vi "FABR-Save Data.vi"(0 "Params":T3={"Stimulus"={"Destination"="", "Rep rate (/sec)"=30.0, "Alternate Polarity"=FALSE, "Duration (ms)"=0.0, "Ramp (ms)"=16.0, "Fs (Hz)"=5.0, "Frame size (s)"=0.0}, "Sequence"={"Freq"={"Start (kHz)"=20.0, "Stop (kHz)"=80.0, "Step (oct)"=5.0, "Skip (oct)"=0.0}, "Level"={"Start (dB)"=20, "Stop (dB)"=80, "Step (dB)"=5}, "Order"=enum."Interleaved"}, "Response"={"Gain"=1.0, "Averages"=0, "Window (ms)"=0.0, "Fs (Hz)"=25000.0, "Save raw"=FALSE}, "Reject"=0.0} {"Sequence"."Level"."Start (dB)" step=5; "Sequence"."Freq"."Start (kHz)" step=5.0; "Response"."Window (ms)" format="%.2f"}, 5 "Path":path, 11 "error in (no error)":errorcluster, 12 "Analysis":T8, 13 "Notes":string) -> (15 "error out":errorcluster)   [LabVIEW 2020]
uses:
  Typedefs/FABR-Analysis State.ctl
  Threshold Estimation VIs/ABR3-Threshold Estimation Result.ctl
  Typedefs/FABR-Parameters.ctl
  Typedefs/FABR-Stimulus.ctl
  Typedefs/FABR-Sequence.ctl
  Typedefs/FABR-Order.ctl
  Typedefs/FABR-Response.ctl
  Typedefs/FABR-Header.ctl
  8c3103e5-e364-4fea-8254-1b02a401fff2.vi
  epl-vi-lib/Utility VIs/Math VIs/LinSpace (x0-dx-npts).vi
  epl-vi-lib/Utility VIs/File IO VIs/Configuration File Wrapper VIs/Config-Read Key (string).vi
  CFTS VIs/CFTS-Globals.vi
panel:
  in  "FAST ABR":T1
  # "Freq X Level X Time"
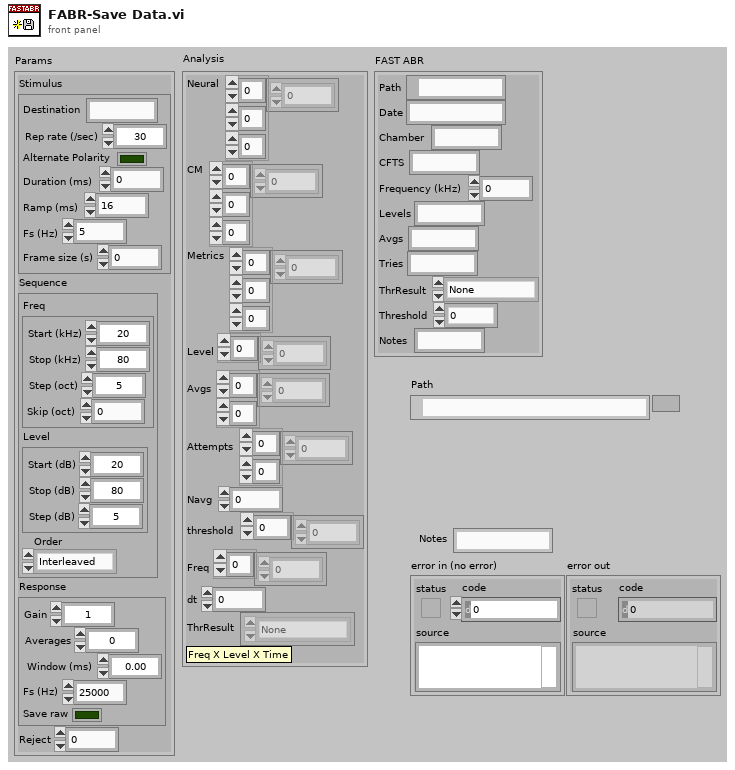
[diagram p1: front panel]
types:
  T1 = typedef "FABR-Header.ctl" = cluster{"Path":path, "Date":string, "Chamber":string, "CFTS":string, "Frequency (kHz)":dbl, "Levels":string, "Avgs":string, "Tries":string, "ThrResult":T2, "Threshold":dbl, "Notes":string}
  T2 = typedef "ABR3-Threshold Estimation Result.ctl" = enum16{"None", "Power", "Sigmoid", "Power (noisy)", "Suprathreshold", "Invalid"}
  T3 = typedef "FABR-Parameters.ctl" = cluster{"Stimulus":T4, "Sequence":T5, "Response":T7, "Reject":dbl}
  T4 = typedef "FABR-Stimulus.ctl" = cluster{"Destination":string, "Rep rate (/sec)":dbl, "Alternate Polarity":bool, "Duration (ms)":dbl, "Ramp (ms)":dbl, "Fs (Hz)":dbl, "Frame size (s)":dbl}
  T5 = typedef "FABR-Sequence.ctl" = cluster{"Freq":cluster{"Start (kHz)":dbl, "Stop (kHz)":dbl, "Step (oct)":dbl, "Skip (oct)":dbl}, "Level":cluster{"Start (dB)":i32, "Stop (dB)":i32, "Step (dB)":i32}, "Order":T6}
  T6 = typedef "FABR-Order.ctl" = enum16{"Interleaved"}
  T7 = typedef "FABR-Response.ctl" = cluster{"Gain":dbl, "Averages":i32, "Window (ms)":sgl, "Fs (Hz)":dbl, "Save raw":bool}
  T8 = typedef "FABR-Analysis State.ctl" = cluster{"Neural":dbl[][][], "CM":dbl[][][], "Metrics":dbl[][][], "Level":dbl[], "Avgs":i32[][], "Attempts":i32[][], "Navg":i32, "threshold":dbl[], "Freq":dbl[], "dt":dbl, "ThrResult":T2[]}
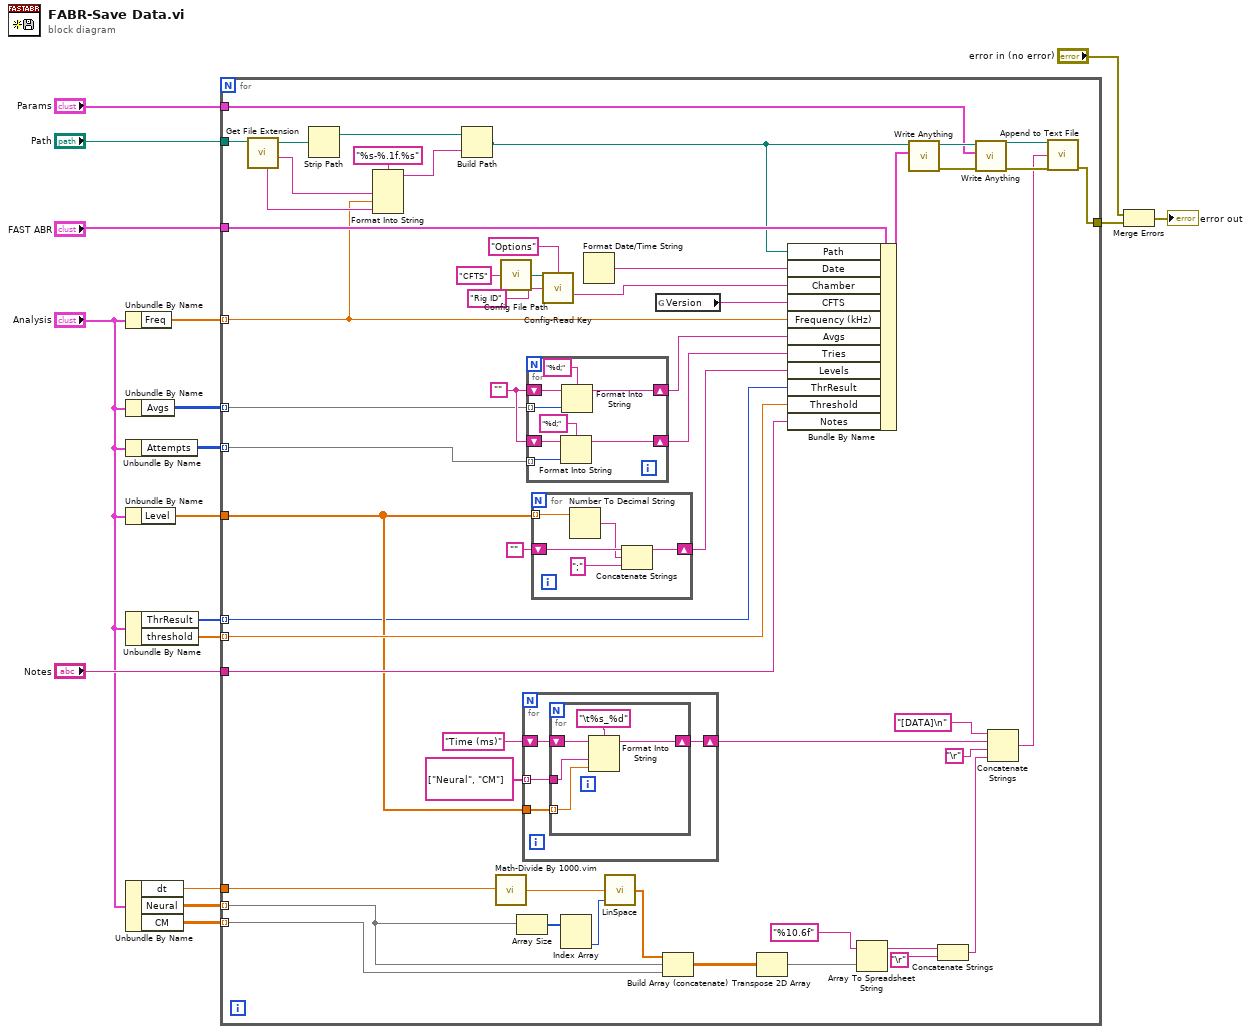
[diagram p0: block diagram]
diagram:
  n1 = Unbundle By Name("Analysis") -> ("Freq"=w12:dbl[])
  n2 = Unbundle By Name("Analysis") -> ("Avgs"=w8:i32[][])
  n3 = Unbundle By Name("Analysis") -> ("Attempts"=w7:i32[][])
  n4 = Unbundle By Name("Analysis") -> ("Level"=w4:dbl[])
  n5 = Unbundle By Name("Analysis") -> ("ThrResult"=w1:T2[], "threshold"=w11:dbl[])
  n6 = Unbundle By Name("Analysis") -> ("dt"=w3:dbl, "Neural"=w10:dbl[][][], "CM"=w9:dbl[][][])
  n7 = for {
    tunnel: "Notes" -> [w35]
    tunnel: [w71] -> w13
    tunnel: "Params" -> [w40]
    tunnel: w12 -> [w18] mode=indexing
    tunnel: w11 -> [w36] mode=indexing
    tunnel: w10 -> [w34] mode=indexing
    tunnel: w9 -> [w33] mode=indexing
    tunnel: w8 -> [w39] mode=indexing
    tunnel: w7 -> [w38] mode=indexing
    tunnel: "FAST ABR" -> [w37]
    tunnel: w4 -> [w31]
    tunnel: w3 -> [w32]
    tunnel: "Path" -> [w27]
    tunnel: w1 -> [w19] mode=indexing
    w44 = ""
    n8 = call <vilib>:"Get File Extension.vi"("file"=w27) -> ("filename without extension"=w24:string, "dup file"=w26:path, "unmodified file extension"=w23:string)  [unwired: 6 in, 2 out]
    n9 = Strip Path(path=w26) -> (stripped path=w22:path)  [unwired: 1 out]
    n10 = Format Into String(format string="%s-%.1f.%s", w24, w18, w23) -> (resulting string=w21:string)  [unwired: 2 in, 1 out]
    n11 = Build Path(base path=w22, name or relative path=w21) -> (appended path=w20:path)
    n12 = call "Math-Divide By 1000.vim"("X"=w32) -> ("1000X"=w56:dbl)
    n13 = call "Config File Path.vi"("AppName"="CFTS") -> ("Default config file name"=w48:path)
    n14 = Array Size(array=w34) -> (size(s)=w55:i32[])
    n15 = for {
      tunnel: w31 -> [w88]
      tunnel: string[] ["Neural", "CM"] -> [w86] mode=indexing
      shift-right: [w85] -> w49
      shift-left: "Time (ms)" -> [w87]
      n16 = for {
        tunnel: w88 -> [w92] mode=indexing
        shift-right: [w90] -> w85
        shift-left: w87 -> [w91]
        tunnel: w86 -> [w89]
        n17 = Format Into String(format string="\t%s_%d", initial string=w91, w89, w92) -> (resulting string=w90:string)  [unwired: 1 in, 1 out]
      }
    }
    n18 = for {
      tunnel: w39 -> [w79] mode=indexing
      tunnel: w38 -> [w75] mode=indexing
      shift-right: [w76] -> w43
      shift-left: w44 -> [w78]
      shift-right: [w73] -> w42
      shift-left: w44 -> [w74]
      n19 = Format Into String(format string="%d;", initial string=w74, w75) -> (resulting string=w73:string)  [unwired: 1 in, 1 out]
      n20 = Format Into String(format string="%d;", initial string=w78, w79) -> (resulting string=w76:string)  [unwired: 1 in, 1 out]
    }
    n21 = for {
      shift-right: [w81] -> w59
      shift-left: "" -> [w84]
      tunnel: w31 -> [w80] mode=indexing
      n22 = Number To Decimal String(number=w80) -> (decimal integer string=w83:string)  [unwired: 1 in]
      n23 = Concatenate Strings(w84, w83, ";") -> (w81:string)
    }
    n24 = call-poly "Config-Read Key.vi"("configuration file path"=w48, "section"="Options", "key"="Rig ID" ("string")) -> ("value"=w45:string)  [unwired: 9 in, 3 out]
    n25 = Index Array(array=w55) -> (element #2=w54:i32)  [unwired: 2 in, 1 out]
    n26 = Format Date/Time String() -> (date/time string=w61:string)  [unwired: 3 in]
    n27 = call-poly "LinSpace.vi"("npts"=w54, "dx"=w56) -> ("Array"=w53:dbl[])  [unwired: 2 in, 1 out]
    n28 = global read "CFTS-Globals.vi" "Version"() -> (w60:string)
    n29 = Build Array (concatenate)(w53, w34, w33) -> (w66:dbl[][])
    n30 = Transpose 2D Array(2D array=w66) -> (transposed array=w57:dbl[][])
    n31 = Bundle By Name(cluster=w37, "Path"=w20, "Date"=w61, "Chamber"=w45, "CFTS"=w60, "Frequency (kHz)"=w18, "Avgs"=w43, "Tries"=w42, "Levels"=w59, "ThrResult"=w19, "Threshold"=w36, "Notes"=w35) -> (w64:T1)
    n32 = Array To Spreadsheet String(array=w57, 3:"%10.6f") -> (spreadsheet string=w68:string)  [unwired: 1 in]
    n33 = call "Write Anything.vi"("Anything"=w64, "Path (dialog)"=w20) -> ("Error Out"=w62:errorcluster, "Path out"=w63:path)  [unwired: 8 in]
    n34 = Concatenate Strings(w68, "\r") -> (w50:string)
    n35 = call "Write Anything.vi"("Error In"=w62, "Anything"=w40, "Path (dialog)"=w63) -> ("Error Out"=w30:errorcluster, "Path out"=w29:path)  [unwired: 7 in]
    n36 = Concatenate Strings("[DATA]\n", w49, "\r", w50) -> (w28:string)
    n37 = call "Append to Text File.vi"("file path"=w29, "text"=w28, "error in (no error)"=w30) -> ("error out"=w71:errorcluster)  [unwired: 11 in, 1 out]
  }
  n38 = Merge Errors("error in (no error)", w13) -> (→"error out":errorcluster)
